vi "ShutDownSequence.vi"(8 "error in":errorcluster, 11 "Cluster":T2) -> (0 "error out":errorcluster)   [LabVIEW 2011]
uses:
  Utilities/controls/ctlSeqFNs_AVTGuppy.ctl
  Utilities/controls/ctlSeqFNs_Scanner.ctl
  Utilities/controls/ctlSeqFNs_CTIOTF.ctl
  Utilities/controls/ctlSeqFNs_Andor.ctl
  Utilities/controls/ctlSeqFNs_Koheras.ctl
  Utilities/controls/ctlSeqFNs_Heidenhain.ctl
  Utilities/controls/ctlSeqFNs_Main.ctl
  <vilib>/userDefined/High Color/IMAQdx.ctl
  Utilities/controls/ctlSeqFNs_PCDeviceInit.ctl
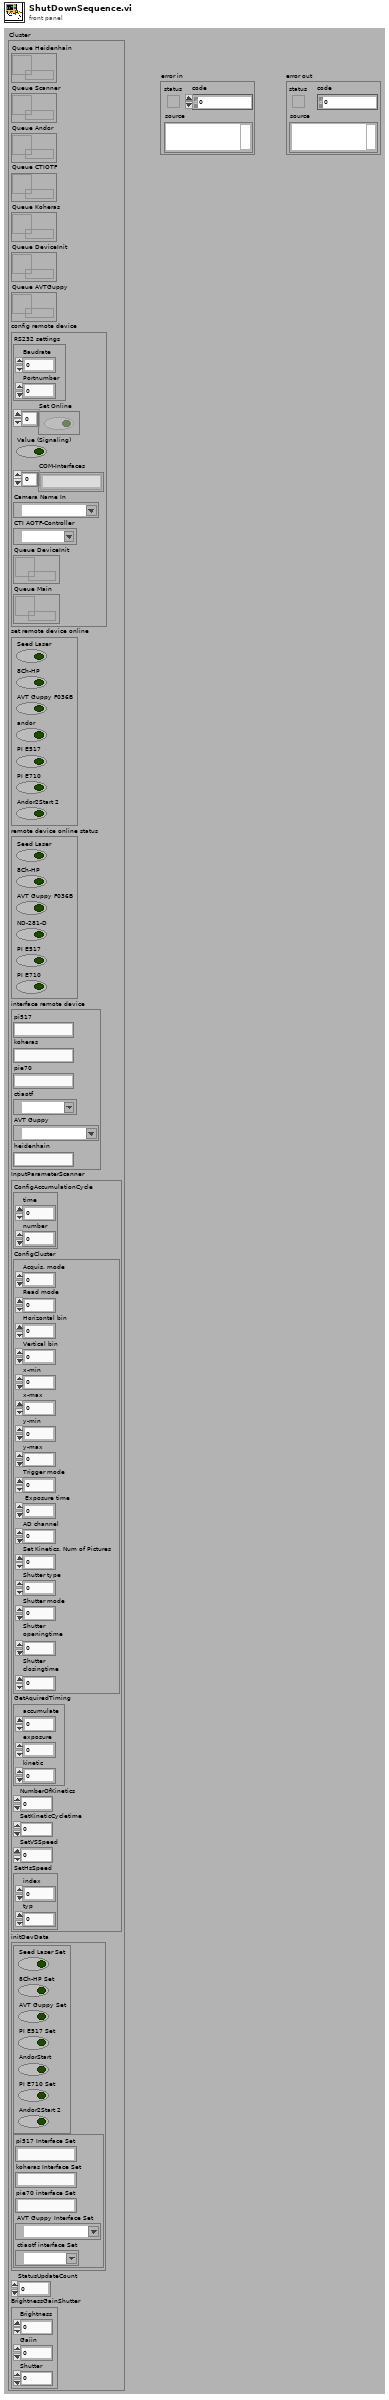
[diagram p1: front panel]
types:
  T1 = typedef "IMAQdx.ctl" = refnum<k21>
  T2 = cluster{"Queue Heidenhain":refnum<queue>, "Queue Scanner":refnum<queue>, "Queue Andor":refnum<queue>, "Queue CTIOTF":refnum<queue>, "Queue Koheras":refnum<queue>, "Queue DeviceInit":refnum<queue>, "Queue AVTGuppy":refnum<queue>, "config remote device":cluster{"RS232 settings":cluster{"Baudrate":u16, "Portnumber":i32}, "Set Online":bool[], "Value (Signaling)":bool, "COM-Interfaces":string[], "Camera Name In":T1, "CTI AOTF-Controller":refnum<visa-resource-name>, "Queue DeviceInit":refnum<queue>, "Queue Main":refnum<queue>}, "set remote device online":cluster{"Seed Laser":bool, "8Ch-HP":bool, "AVT Guppy F036B":bool, "andor":bool, "PI E517":bool, "PI E710":bool, "Andor2Start 2":bool}, "remote device online status":cluster{"Seed Laser":bool, "8Ch-HP":bool, "AVT Guppy F036B":bool, "ND-281-D":bool, "PI E517":bool, "PI E710":bool}, "interface remote device":cluster{"pi517":string, "koheras":string, "pie70":string, "ctiaotf":refnum<visa-resource-name>, "AVT Guppy":T1, "heidenhain":string}, "InputParameterScanner":cluster{"ConfigAccumulationCycle":cluster{"time":sgl, "number":i32}, "ConfigCluster":cluster{"Acquis. mode":u16, "Read mode":u16, "Horizontal bin":i32, "Vertical bin":i32, "x-min":i32, "x-max":i32, "y-min":i32, "y-max":i32, "Trigger mode":u16, " Exposure time":sgl, "AD channel":i32, "Set Kinetics, Num of Pictures":i32, "Shutter type":u16, "Shutter mode":u16, "Shutter\nopeningtime":i32, "Shutter\nclosingtime":i32}, "GetAquiredTiming":cluster{"accumulate":sgl, "exposure":sgl, "kinetic":sgl}, "NumberOfKinetics":i32, "SetKineticCycletime":sgl, "SetVSSpeed":i32, "SetHsSpeed":cluster{"index":i32, "typ":i32}}, "initDevData":cluster{cluster{"Seed Laser Set":bool, "8Ch-HP Set":bool, "AVT Guppy Set":bool, "PI E517 Set":bool, "AndorStart":bool, "PI E710 Set":bool, "Andor2Start 2":bool}, cluster{"pi517 Interface Set":string, "koheras Interface Set":string, "pie70 interface Set":string, "AVT Guppy Interface Set":T1, "ctiaotf interface Set":refnum<visa-resource-name>}}, "StatusUpdateCount":dbl, "BrightnessGainShutter":cluster{"Brightness":i32, "Gaiin":i32, "Shutter":i32}}
  T3 = typedef "ctlSeqFNs_Heidenhain.ctl" = enum16{"ERROR", "INIT", "Initialization", "Configuration", "Measurement", "Shutdown", "IDLE", "EXIT"}
  T4 = typedef "ctlSeqFNs_Koheras.ctl" = enum16{"ERROR", "INIT", "Initialization", "Configuration", "Measurement", "Shutdown", "IDLE", "EXIT"}
  T5 = typedef "ctlSeqFNs_Andor.ctl" = enum16{"ERROR", "INIT", "Initialization", "Configuration", "Measurement", "Shutdown", "IDLE", "EXIT"}
  T6 = typedef "ctlSeqFNs_CTIOTF.ctl" = enum16{"ERROR", "INIT", "Initialization", "Configuration", "Measurement", "Shutdown", "IDLE", "EXIT"}
  T7 = typedef "ctlSeqFNs_Scanner.ctl" = enum16{"ERROR", "INIT", "Initialization", "Configuration", "Measurement", "Shutdown", "IDLE", "EXIT"}
  T8 = typedef "ctlSeqFNs_AVTGuppy.ctl" = enum16{"ERROR", "INIT", "Initialization", "Configuration", "Measurement", "Shutdown", "IDLE", "EXIT"}
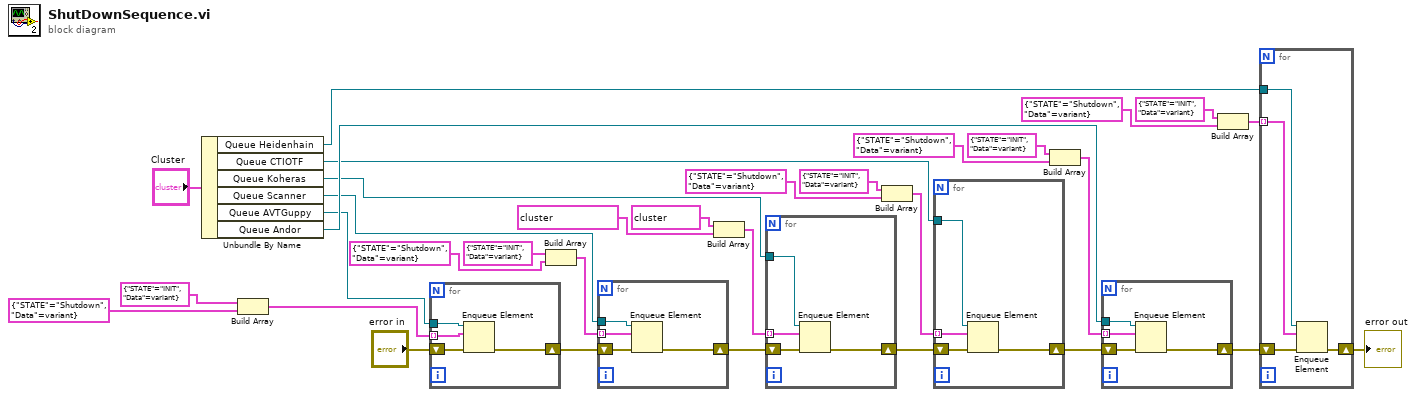
[diagram p0: block diagram]
diagram:
  n1 = Unbundle By Name("Cluster") -> ("Queue Heidenhain"=w1:refnum<queue>, "Queue CTIOTF"=w18:refnum<queue>, "Queue Koheras"=w16:refnum<queue>, "Queue Scanner"=w12:refnum<queue>, "Queue AVTGuppy"=w10:refnum<queue>, "Queue Andor"=w21:refnum<queue>)
  n2 = Build Array(cluster{"STATE":T8, "Data":variant} {"STATE"=enum."INIT", "Data"=variant} ("element"), cluster{"STATE":T8, "Data":variant} {"STATE"=enum."Shutdown", "Data"=variant} ("element")) -> (w9:cluster{"STATE":T8, "Data":variant}[])
  n3 = for {
    tunnel: w10 -> [w36]
    shift-right: [w34] -> w11
    shift-left: "error in" -> [w35]
    tunnel: w9 -> [w33] mode=indexing
    n4 = Enqueue Element(queue=w36, element=w33, error in (no error)=w35) -> (error out=w34:errorcluster)  [unwired: 1 in, 2 out]
  }
  n5 = Build Array(cluster{"STATE":T7, "Data":variant} {"STATE"=enum."INIT", "Data"=variant} ("element"), cluster{"STATE":T7, "Data":variant} {"STATE"=enum."Shutdown", "Data"=variant} ("element")) -> (w13:cluster{"STATE":T7, "Data":variant}[])
  n6 = for {
    tunnel: w12 -> [w40]
    shift-right: [w38] -> w15
    shift-left: w11 -> [w39]
    tunnel: w13 -> [w37] mode=indexing
    n7 = Enqueue Element(queue=w40, element=w37, error in (no error)=w39) -> (error out=w38:errorcluster)  [unwired: 1 in, 2 out]
  }
  n8 = Build Array(cluster{"Data":variant, "FGV_Control":T4} {"Data"=variant, "FGV_Control"=enum."INIT"} ("element"), cluster{"Data":variant, "FGV_Control":T4} {"Data"=variant, "FGV_Control"=enum."Shutdown"} ("element")) -> (w17:cluster{"Data":variant, "FGV_Control":T4}[])
  n9 = for {
    tunnel: w16 -> [w44]
    shift-right: [w42] -> w20
    shift-left: w15 -> [w43]
    tunnel: w17 -> [w41] mode=indexing
    n10 = Enqueue Element(queue=w44, element=w41, error in (no error)=w43) -> (error out=w42:errorcluster)  [unwired: 1 in, 2 out]
  }
  n11 = Build Array(cluster{"STATE":T6, "Data":variant} {"STATE"=enum."INIT", "Data"=variant} ("element"), cluster{"STATE":T6, "Data":variant} {"STATE"=enum."Shutdown", "Data"=variant} ("element")) -> (w19:cluster{"STATE":T6, "Data":variant}[])
  n12 = for {
    tunnel: w18 -> [w48]
    shift-right: [w46] -> w22
    shift-left: w20 -> [w47]
    tunnel: w19 -> [w45] mode=indexing
    n13 = Enqueue Element(queue=w48, element=w45, error in (no error)=w47) -> (error out=w46:errorcluster)  [unwired: 1 in, 2 out]
  }
  n14 = Build Array(cluster{"STATE":T5, "Data":variant} {"STATE"=enum."INIT", "Data"=variant} ("element"), cluster{"STATE":T5, "Data":variant} {"STATE"=enum."Shutdown", "Data"=variant} ("element")) -> (w25:cluster{"STATE":T5, "Data":variant}[])
  n15 = for {
    tunnel: w21 -> [w52]
    shift-right: [w50] -> w4
    shift-left: w22 -> [w51]
    tunnel: w25 -> [w49] mode=indexing
    n16 = Enqueue Element(queue=w52, element=w49, error in (no error)=w51) -> (error out=w50:errorcluster)  [unwired: 1 in, 2 out]
  }
  n17 = Build Array(cluster{"STATE":T3, "Data":variant} {"STATE"=enum."INIT", "Data"=variant} ("element"), cluster{"STATE":T3, "Data":variant} {"STATE"=enum."Shutdown", "Data"=variant} ("element")) -> (w5:cluster{"STATE":T3, "Data":variant}[])
  n18 = for {
    tunnel: w1 -> [w56]
    shift-right: [w54] -> w3
    shift-left: w4 -> [w55]
    tunnel: w5 -> [w53] mode=indexing
    n19 = Enqueue Element(queue=w56, element=w53, error in (no error)=w55) -> (error out=w54:errorcluster)  [unwired: 1 in, 2 out]
  }
  "error out" <- w3
